vi "Dice game.vi"() -> ()   [LabVIEW 2014]
panel:
  out "B average":dbl
  out "A average":dbl
  out "Tie game rate":dbl
  out "B win rate":dbl
  out "A win rate":dbl
  out "player2 past":T1
  out "player1 past":T1
  out "Result":string
  out "Times":i32
  out "Waveform Chart":cluster{dbl, dbl, dbl}(graph)
  out "Tie game":dbl
  out "B win":dbl
  out "A win":dbl
  out "B":dbl
  in  "Roll Button 2":bool
  out "A":dbl
  in  "Roll Button":bool
  in  "STOP Button":bool
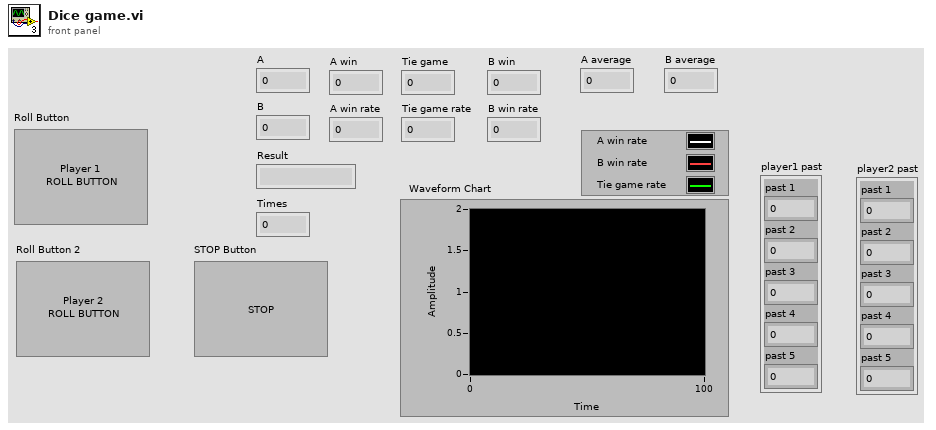
[diagram p1: front panel]
types:
  T1 = cluster{"past 1":dbl, "past 2":dbl, "past 3":dbl, "past 4":dbl, "past 5":dbl}
  T2 = cluster{"Dice":dbl, "Dice":dbl, "Dice":dbl, "Dice":dbl, "Dice":dbl}
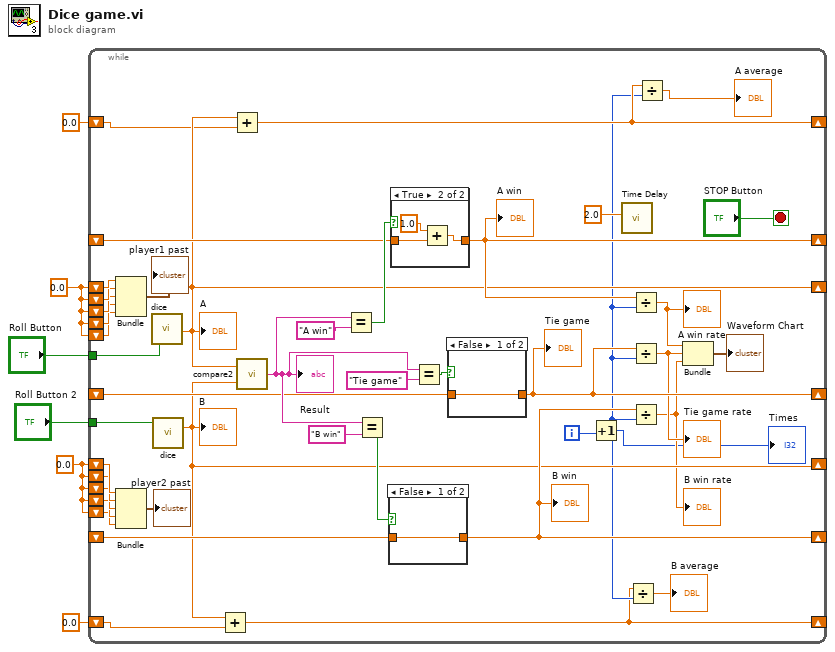
[diagram p0: block diagram]
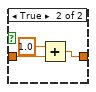
[diagram p2: hidden frame]
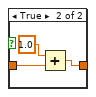
[diagram p3: hidden frame]
diagram:
  w3 = 0.0 ("Dice")
  w4 = 0.0 ("Dice")
  n1 = while {
    tunnel: "Roll Button" -> [w41]
    tunnel: "Roll Button 2" -> [w40]
    shift-right: [w37] -> _
    shift-left: _ -> [w36]
    shift-right: [w21] -> _
    shift-left: _ -> [w35]
    shift-right: [w19] -> _
    shift-left: _ -> [w34]
    shift-right: [w17] -> _
    shift-left: w4 -> [w33]
    shift-left: w4 -> [w32]
    shift-left: w4 -> [w31]
    shift-left: w4 -> [w30]
    shift-left: w4 -> [w29]
    shift-right: [w15] -> _
    shift-left: w3 -> [w27]
    shift-left: w3 -> [w26]
    shift-left: w3 -> [w25]
    shift-left: w3 -> [w24]
    shift-left: w3 -> [w23]
    shift-right: [w9] -> _
    shift-left: 0.0 -> [w16]
    shift-right: [w7] -> _
    shift-left: 0.0 -> [w14]
    i -> [w20]
    stop <- "STOP Button" stop-if-true
    n2 = Bundle("Dice"=w33, "Dice"=w32, "Dice"=w31, "Dice"=w30, "Dice"=w29) -> (→"player1 past":T2)  [unwired: 1 in]
    n3 = Bundle("Dice"=w27, "Dice"=w26, "Dice"=w25, "Dice"=w24, "Dice"=w23) -> (→"player2 past":T2)  [unwired: 1 in]
    n4 = call "dice.vi"("PUSH Button"=w41) -> ("Dice"=w17:dbl)  [unwired: 1 in]
    "A" <- w17
    n5 = call "dice.vi"("PUSH Button"=w40) -> ("Dice"=w15:dbl)  [unwired: 1 in]
    "B" <- w15
    n6 = Add(x=w15, y=w14) -> (x+y=w7:dbl)
    n7 = Add(x=w17, y=w16) -> (x+y=w9:dbl)
    n8 = call "compare2.vi"("B"=w15, "A"=w17) -> ("String"=w43:string)
    "Result" <- w43
    n9 = Equal?(x=w43, y="A win") -> (x = y?=w39:bool)
    n10 = Equal?(x=w43, y="B win") -> (x = y?=w18:bool)
    n11 = case shown="False" w18 {
      tunnel: w34 -> [w50 w51]
      tunnel: [w50 w52] -> w19
      frame False {
      }
      frame True {
        n12 = Add(x=1.0, y=w51) -> (x+y=w52:dbl)
      }
    }
    "B win" <- w19
    n13 = case shown="True" w39 {
      tunnel: w36 -> [w58 w59]
      tunnel: [w58 w60] -> w37
      frame False {
      }
      frame True {
        n14 = Add(x=1.0, y=w59) -> (x+y=w60:dbl)
      }
    }
    "A win" <- w37
    n15 = Equal?(x=w43, y="Tie game") -> (x = y?=w38:bool)
    n16 = case shown="False" w38 {
      tunnel: w35 -> [w54 w55]
      tunnel: [w54 w56] -> w21
      frame False {
      }
      frame True {
        n17 = Add(x=1.0, y=w55) -> (x+y=w56:dbl)
      }
    }
    "Tie game" <- w21
    n18 = Increment(x=w20) -> (x+1=w8:i32)
    "Times" <- w8
    n19 = call "Time Delay"("Delay Time (s)"=2.0) -> ()  [unwired: 10 in, 1 out]
    n20 = Divide(x=w7, y=w8) -> (x/y=→"B average":dbl)
    n21 = Divide(x=w37, y=w8) -> (x/y=w46:dbl)
    "A win rate" <- w46
    n22 = Divide(x=w21, y=w8) -> (x/y=w12:dbl)
    "Tie game rate" <- w12
    n23 = Divide(x=w19, y=w8) -> (x/y=w11:dbl)
    "B win rate" <- w11
    n24 = Divide(x=w9, y=w8) -> (x/y=→"A average":dbl)
    n25 = Bundle(w46, w12, w11) -> (→"Waveform Chart":cluster{dbl, dbl, dbl})  [unwired: 1 in]
  }
